vi "NOx_Example_FPGA.vi"() -> ()   [LabVIEW 2011]
uses:
  <vilib>/rvi/eio/common/nirviEmuTemplateMethod_errors.vi
  <vilib>/eio/EIOMethodNode/EIOMethodNode.xnode
  <vilib>/eio/EIONode/EIONode.xnode
  <vilib>/LabVIEW Targets/FPGA/RIO/nicrio_985x_controls.llb/CAN_IO_Frame Cluster.ctl
  <vilib>/LabVIEW Targets/FPGA/RIO/nicrio_985x_controls.llb/CAN_IO_Frame Type.ctl
panel:
  out "NOxSensorData 2":T1={"NOx (bits)"=0, "O2 (bits)"=0, "Sensor Supply Status"=3, "Sensor Temperature Status"=12, "NOx Signal Status"=48, "O2 Signal Status"=192, "Heater Mode Status"=96, "Heater Circuit Status"=31, "NOx Circuit Status"=31, "O2 Circuit Status"=31, "NOx Sensor Module Present"=FALSE} {"Heater Mode Status" items=["AUTO MODE"=0, "HEATUP SLOPE 3 OR 4"=32, "HEATUP SLOPE 1 OR 2"=64, "HEATER OFF / PREHEAT"=96]; "O2 Circuit Status" items=["OPEN WIRE"=3, "SHORT CIRCUIT"=5, "NO ERROR"=31]; "NOx Circuit Status" items=["OPEN WIRE"=3, "SHORT CIRCUIT"=5, "NO ERROR"=31]; "Heater Circuit Status" items=["OPEN WIRE"=3, "SHORT CIRCUIT"=5, "NO ERROR"=31]; "Sensor Temperature Status" items=["NOT AT TEMPERATURE"=0, "AT TEMPERATURE"=4, "ERROR"=8, "NOT AVAILABLE"=12]; "O2 Signal Status" items=["NOT VALID"=0, "VALID"=64, "ERROR"=128, "NOT AVAILABLE"=192]; "NOx Signal Status" items=["NOT VALID"=0, "VALID"=16, "ERROR"=32, "NOT AVAILABLE"=48]; "Sensor Supply Status" items=["NOT IN RANGE", "SUPPLY IN RANGE", "ERROR", "NOT AVAILABLE"]}
  in  "RxID 2":u32=418385489 format="%08x"
  in  "Sensor 2 Enable":bool
  out "RxID Actual":u32 format="%08x"
  out "NOxSensorData 1":T1={"NOx (bits)"=0, "O2 (bits)"=0, "Sensor Supply Status"=3, "Sensor Temperature Status"=12, "NOx Signal Status"=48, "O2 Signal Status"=192, "Heater Mode Status"=96, "Heater Circuit Status"=31, "NOx Circuit Status"=31, "O2 Circuit Status"=31, "NOx Sensor Module Present"=FALSE} {"Heater Mode Status" items=["AUTO MODE"=0, "HEATUP SLOPE 3 OR 4"=32, "HEATUP SLOPE 1 OR 2"=64, "HEATER OFF / PREHEAT"=96]; "O2 Circuit Status" items=["OPEN WIRE"=3, "SHORT CIRCUIT"=5, "NO ERROR"=31]; "NOx Circuit Status" items=["OPEN WIRE"=3, "SHORT CIRCUIT"=5, "NO ERROR"=31]; "Heater Circuit Status" items=["OPEN WIRE"=3, "SHORT CIRCUIT"=5, "NO ERROR"=31]; "Sensor Temperature Status" items=["NOT AT TEMPERATURE"=0, "AT TEMPERATURE"=4, "ERROR"=8, "NOT AVAILABLE"=12]; "O2 Signal Status" items=["NOT VALID"=0, "VALID"=64, "ERROR"=128, "NOT AVAILABLE"=192]; "NOx Signal Status" items=["NOT VALID"=0, "VALID"=16, "ERROR"=32, "NOT AVAILABLE"=48]; "Sensor Supply Status" items=["NOT IN RANGE", "SUPPLY IN RANGE", "ERROR", "NOT AVAILABLE"]}
  in  "CAN0 Restart":bool
  in  "TxID":u32=419356416 format="%08x"
  in  "RxID 1":u32=418385746 format="%08x"
  in  "Sensor 1 Enable":bool
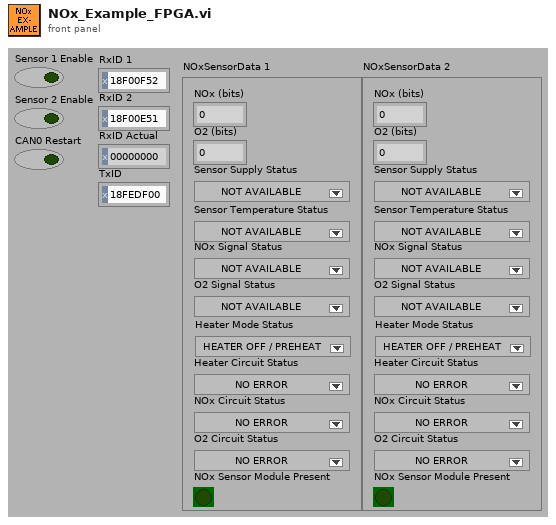
[diagram p1: front panel]
types:
  T1 = cluster{"NOx (bits)":u16, "O2 (bits)":u16, "Sensor Supply Status":u8, "Sensor Temperature Status":u8, "NOx Signal Status":u8, "O2 Signal Status":u8, "Heater Mode Status":u8, "Heater Circuit Status":u8, "NOx Circuit Status":u8, "O2 Circuit Status":u8, "NOx Sensor Module Present":bool}
  T2 = typedef "CAN_IO_Frame Cluster.ctl" = cluster{"timestamp high":u32, "timestamp low":u32, "identifier":u32, "type":T3, "info A":u8, "info B":u8, "data length":u8, "data":u8[]}
  T3 = typedef "CAN_IO_Frame Type.ctl" = enum8{"Data Frame", "Remote Frame", "(reserved)", "(reserved) ", "(reserved)  ", "(reserved)   ", "Bus Error", "Transceiver Fault"}
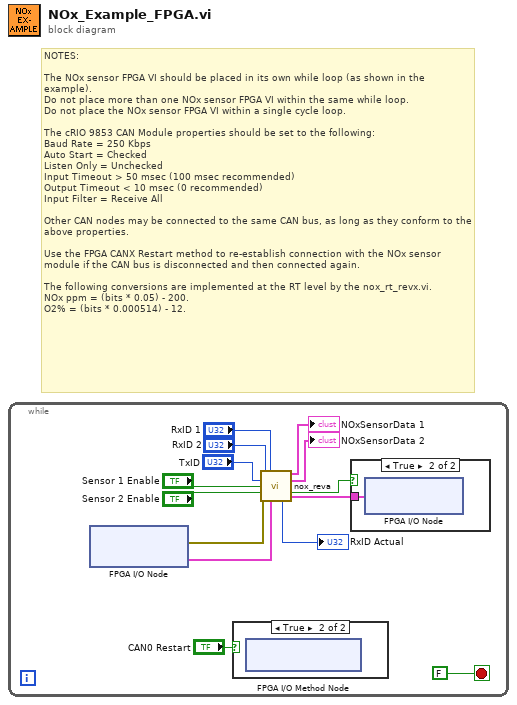
[diagram p0: block diagram]
diagram:
  # "NOTES:\n\nThe NOx sensor FPGA VI should be placed in its own while loop (as shown in the example).  \nDo not place more than one NOx sensor FPGA VI within the same while loop.\nDo not place the NOx sensor FPGA VI within a single cycle loop.\n\nThe cRIO 9853 CAN Module properties should be set to the following:\nBaud Rate = 250 Kbps \nAuto Start = Checked\nListen Only = Unchecked\nInput Timeout > 50 msec (100 msec recommended)\nOutput Timeout < 10 msec (0 recommended)\nInput Filter = Receive All\n\nOther CAN nodes may be connected to the same CAN bus, as long as they conform to the above properties.\n\nUse the FPGA CANX Restart method to re-establish connection with the NOx sensor module if the CAN bus is disconnected and then connected again.\n\nThe following conversions are implemented at the RT level by the nox_rt_revx.vi.\nNOx ppm = (bits * 0.05) - 200.\nO2% = (bits * 0.000514) - 12."
  n1 = while {
    stop <- FALSE stop-if-true
    n2 = xnode "FPGA I/O Node"() -> ("error out"=w13:errorcluster, "NOxCANR"=w12:T2)  [unwired: 2 in, 1 out]
    n3 = case shown="True" "CAN0 Restart" {
      frame False {
      }
      frame True {
        n4 = xnode "FPGA I/O Method Node"() -> ()  [unwired: 1 in, 1 out]
      }
    }
    n5 = call <vilib>:"nox_reva.vi"("RxID 2"="RxID 2", "RxID 1"="RxID 1", "TxID"="TxID", "Sensor1Enable"="Sensor 1 Enable", "Sensor2Enable"="Sensor 2 Enable", "CAN Error In"=w13, "CAN Data In"=w12) -> ("NOxSensorData 1"=→"NOxSensorData 1":T1, "NOxSensorData 2"=→"NOxSensorData 2":T1, "Update CAN Out"=w10:bool, "RxIDActual"=→"RxID Actual":u32, "CAN Data Out"=w9:T2)  [unwired: 4 out]
    n6 = case shown="True" w10 {
      tunnel: w9 -> [_ w15]
      frame False {
      }
      frame True {
        n7 = xnode "FPGA I/O Node"("NOxCANR"=w15) -> ()  [unwired: 1 in, 1 out]
      }
    }
  }
